vi "About LabActor.vi"   [LabVIEW 2016]
panel:
  # "LabActor Framework"
  # "© 2012-2017\n\nFedor F. Balakirev\nfbalakirev@gmail.com"
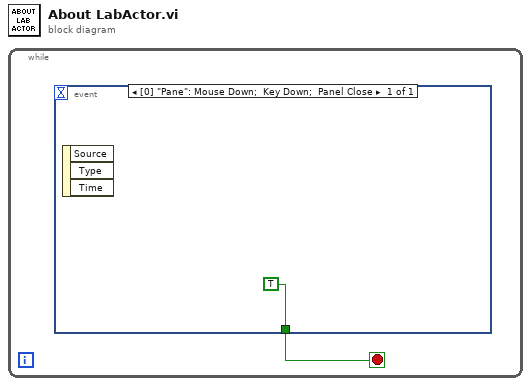
[diagram p0: block diagram]
diagram:
  n1 = while {
    stop <- w1 stop-if-true
    n2 = event shown="[0] \"Pane\": Mouse Down;  Key Down;  Panel Close" {
      selector: _ -> [_]
      dyn-events: _ -> [_]
      timeout: _ -> [_]
      tunnel: [TRUE] -> w1
      event Mouse Down; Key Down; Panel Close {
        n3 = event-data() -> ()  [unwired: 1 in, 3 out]
      }
    }
  }
